vi "Kinesis - MST602 MNA601 - Two Axis Scan.vi"() -> ()   [LabVIEW 2012]
uses:
  U:/Kinesis LabVIEW Website Examples/Thorlabs.MotionControl.Controls.dll
  Thorlabs.MotionControl.Controls.dll
  U:/Kinesis LabVIEW Website Examples/Thorlabs.MotionControl.ModularRackCLI.dll
  Thorlabs.MotionControl.ModularRackCLI.dll
  U:/Kinesis LabVIEW Website Examples/Thorlabs.MotionControl.GenericNanoTrakCLI.dll
  Thorlabs.MotionControl.GenericNanoTrakCLI.dll
  U:/Kinesis LabVIEW Website Examples/Thorlabs.MotionControl.GenericMotorCLI.dll
  Thorlabs.MotionControl.GenericMotorCLI.dll
panel:
  in  "MNA601 Serial Number":string
  in  "MST602 Serial Number":string
  in  "SelectedRange":i32(ring)=3 items=["TIA_Range1_3NA"=3, "TIA_Range2_10NA"=4, "TIA_Range3_30NA"=5, "TIA_Range4_100NA"=6, "TIA_Range5_300NA"=7, "TIA_Range6_1MUA"=8, "TIA_Range7_3MUA"=9, "TIA_Range8_10MUA"=10, "TIA_Range9_30MUA"=11, "TIA_Range10_100MUA"=12, "TIA_Range11_300MUA"=13, "TIA_Range12_1MA"=14, "TIA_Range13_3MA"=15, "TIA_Range14_10MA"=16]
  in  "?":bool
  in  "Num Of Steps":i32=50
  in  "Scale":sgl=0.25 format="%.2f"
  in  "ModularStepperControl Ch.2":refnum<k24>(container)
  in  "ModularStepperControl Ch.1":refnum<k24>(container)
  out "Error":errorcluster
  in  "ModularNanoTrakControl":refnum<k24>(container)
  # "Thorlabs Hardware: \nMST602 Rack Module 2-Ch Stepper Motor Controller \nhttps://www.thorlabs.com/newgrouppage9.cfm?objectgroup_id=1186\n\nMNA601 Rack Module Fiber Auto-alignment Module\nhttps://www.thorlabs.com/newgrouppage9.cfm?objectgroup_id=1187\n\nDescription: The below VI will enable you to connect to a MNA601 & MST602. This VI will initiate a simple 2D raster scan of a Stepper Motor actuated stage. An example of this application setup is pictured whereby the MST602 is driving will drive the internal X & Z piezo blocks of a MAX381 stage. The MAX381 stage is holding an optical fibre aligned to a waveguide in series with secondary receiving fibre via use of Thorlabs flexure stage holder accessories. The secondary fibre is mounted to a secondary co-located MAX302 stage. This fibre is connected to the Optical Input of the MNA601 controller.\n\nThe motorised raster scan will stop either when the max number of steps have been reached or the user selected TIA Range of the MNA601 has been reached, indicating that the MNA601 is reading sufficient photocurrent from the fibre-copupling system. This signifies an \"optimised throughput\" in the system. The MNA601 is defaulted to 'Latch' mode as the MNA601 HV Outputs are not in use.\n\nInstructions: \n1) Connect a MNA601 & MST602 to MMR601 as per the respective product user manuals. These can be connected to any bay in the MMR601 rack.\n2) Enter the module serial numbers below.\n3) Enter the Scan parameters, as well as the exitting TIA Range.\n4) To run the VI, click the run button in the LabVIEW Toolbar.\n5) Once running, the Kinesis UIs will initialise & the VI will wait for you to assign the correct motor types. This can be done by selecting the actuator type on the Kinesis device name on the UI panel & then click 'ACTUATOR SELECTED'\n4) The VI will exit when either the required TIA Range has been reached or the scan has completed."
  # "Notes:"
  # "- Ensure that the appropriate .DLLs are copied into your Project Folder. Check that the correct bit type are used depending on your version of LabVIEW\ni.e. 32-bit or 64-bit.\n\n\n\n\n\n\n\n\n\n\n\n\n\n\n- Open the example VI through the LabVIEW Project Explorer to correctly load the User Interface from Thorlabs.MotionControl.Controls.dll."
  # "Example Image of .NET Controller - VI opened via Project Explorer/ not opened via Project Explorer"
  # "VI Not Opened via Project Explorer"
  # "VI Opened via Project Explorer"
  # "- To explore the range of methods available, please visit the .NET API, included with your Kinesis software.\n\n- For tips on building your own VIs with Thorlabs Motion Control Hardware, please see our LabVIEW Guide here.\nhttps://www.thorlabs.com/newgrouppage9.cfm?objectgroup_id=10285"
  # "52808314"
  # "51810791"
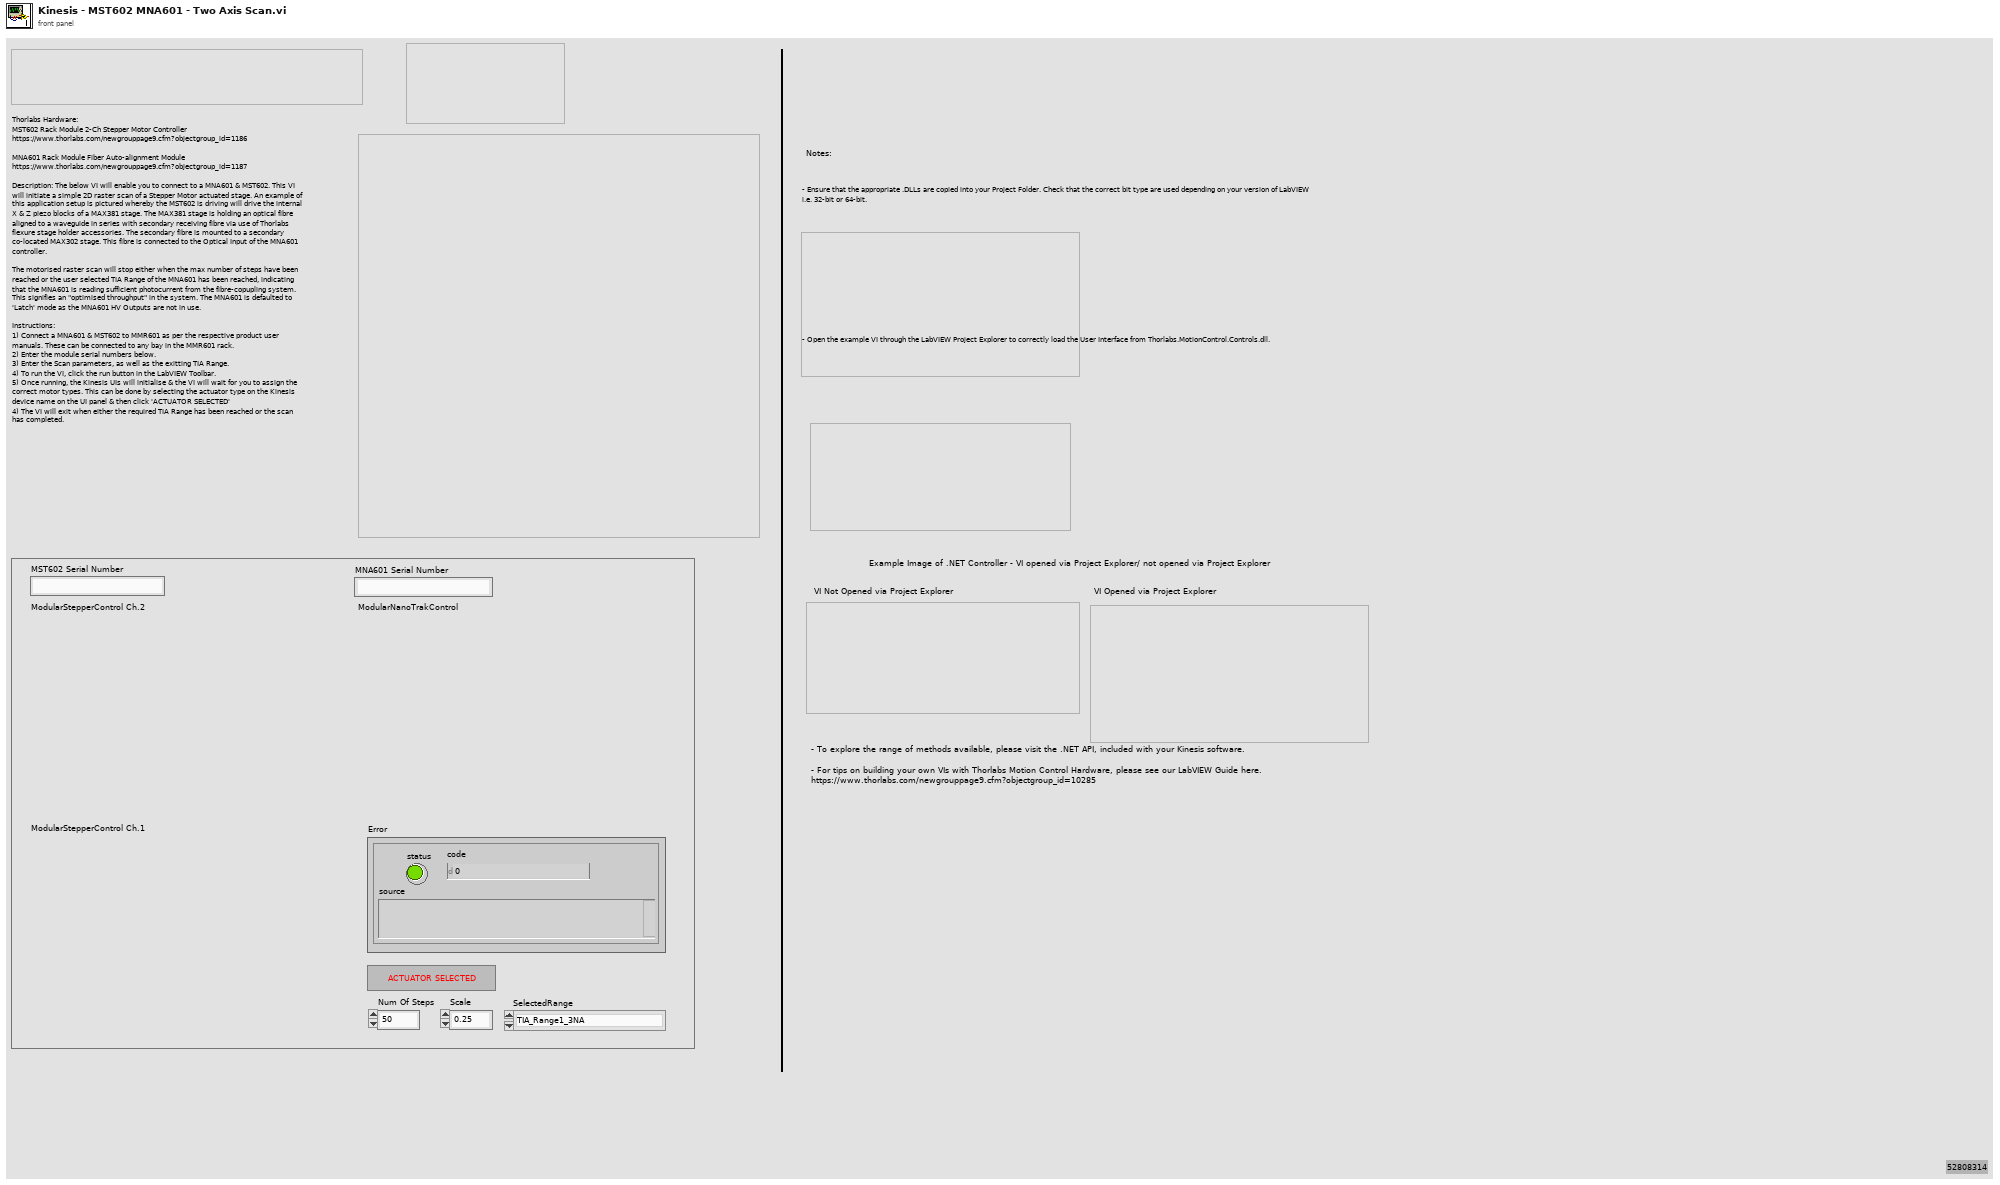
[diagram p1: front panel]
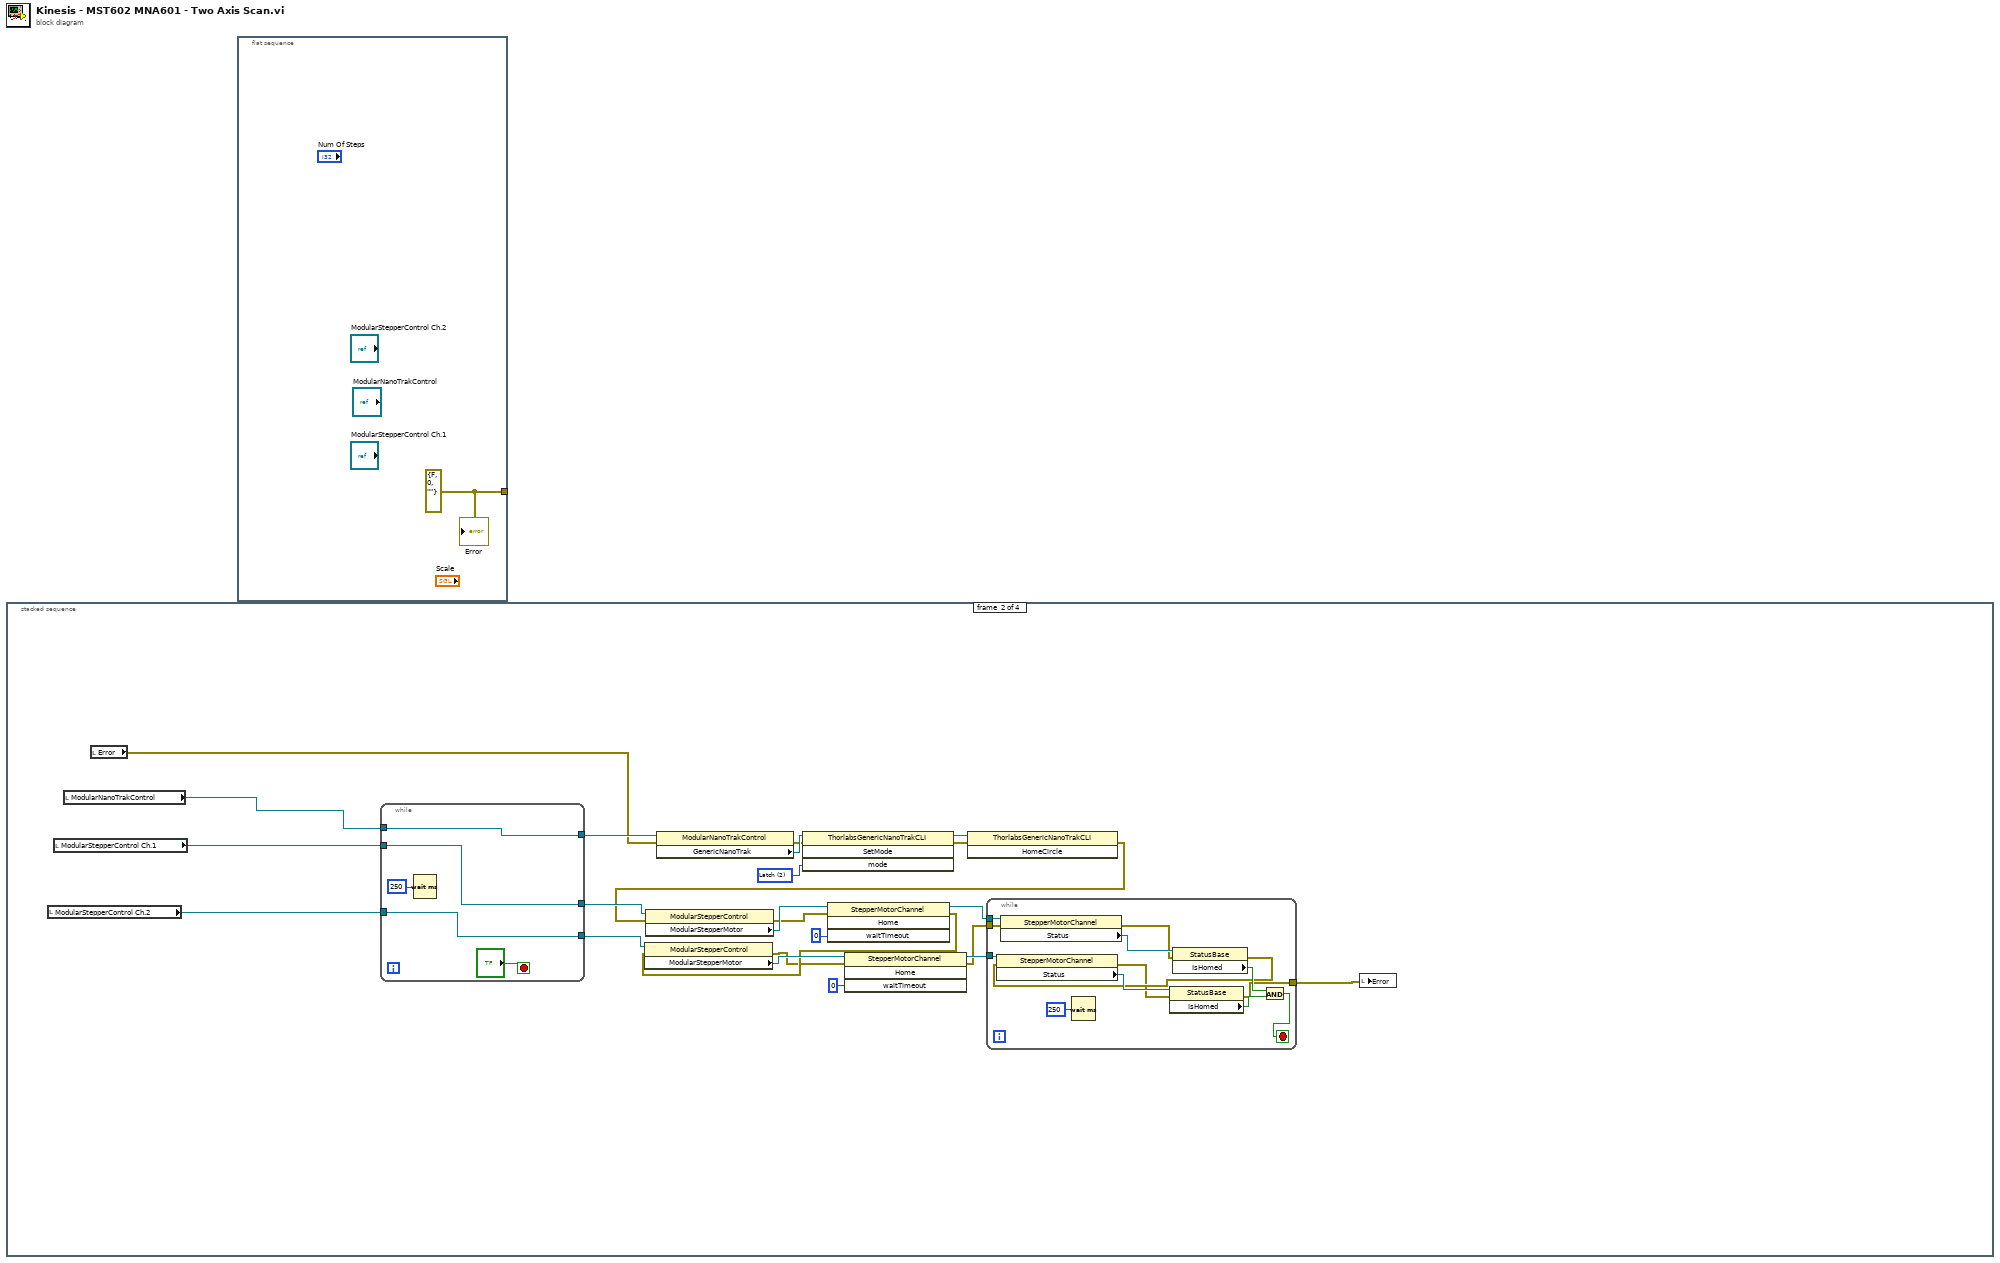
[diagram p0: block diagram]
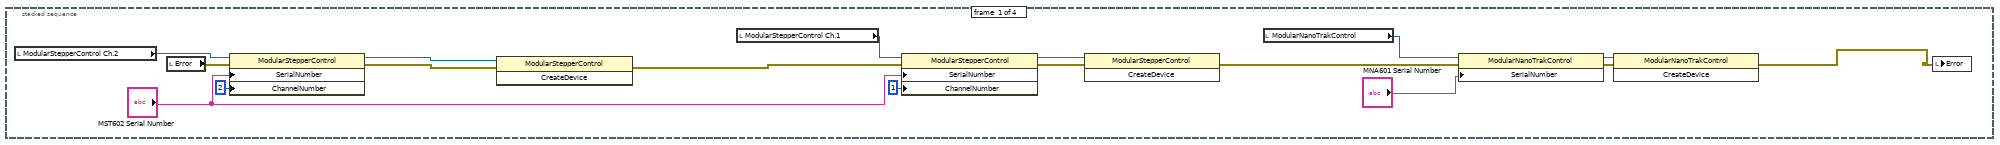
[diagram p2: hidden frame]
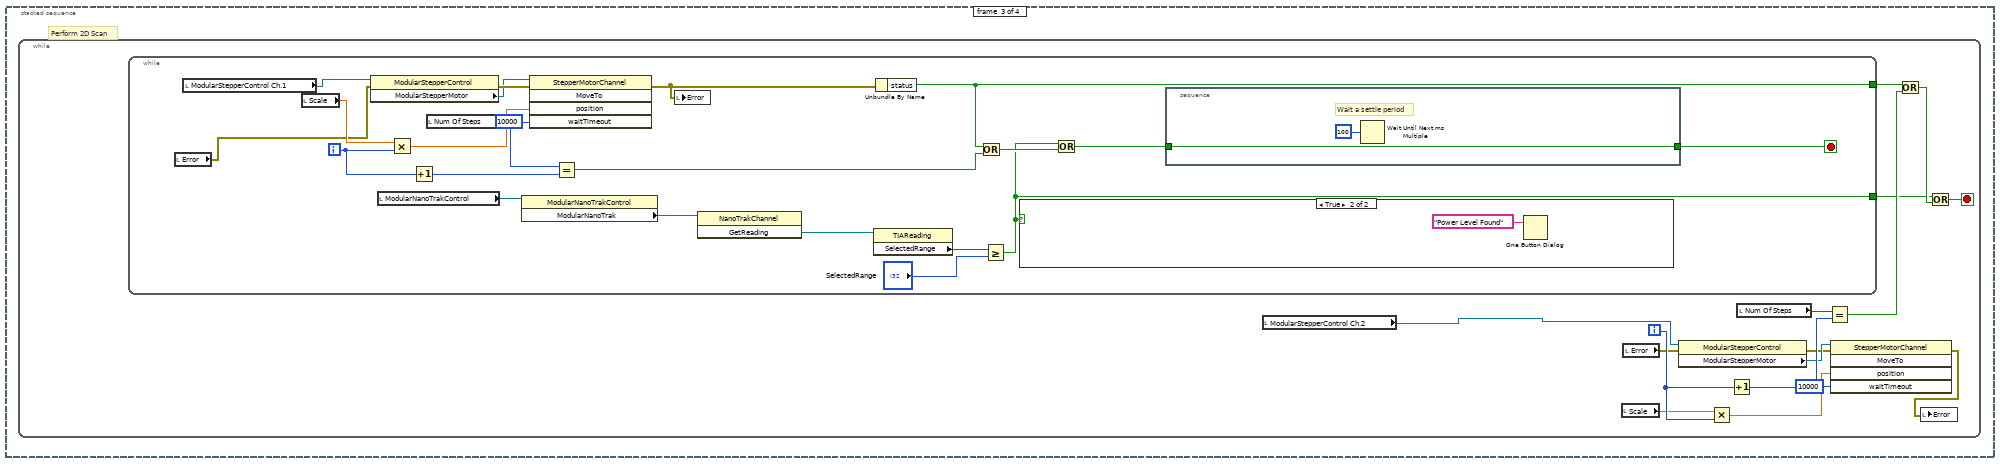
[diagram p3: hidden frame]
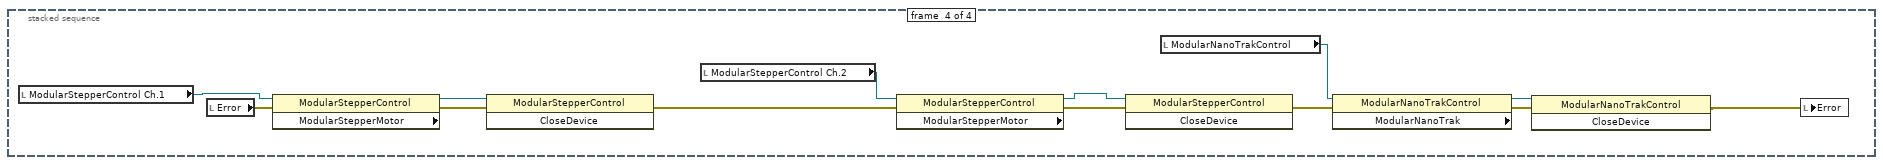
[diagram p5: hidden frame]
diagram:
  n1 = stacked-sequence {
    frame #0 {
      n2 = local read "ModularStepperControl Ch.2"() -> (w7:refnum<k24>)
      n3 = local read "Error"() -> (w14:errorcluster)
      n4 = property class="ModularStepperControl"(reference=w7, error in=w14, "SerialNumber"="MST602 Serial Number", "ChannelNumber"=2) -> (reference out=w17:refnum<k24>, error out=w16:errorcluster)
      n5 = invoke class="ModularStepperControl" method="CreateDevice"(reference=w17, error in=w16) -> (error out=w4:errorcluster)  [unwired: 1 in, 2 out]
      n6 = local read "ModularStepperControl Ch.1"() -> (w6:refnum<k24>)
      n7 = property class="ModularStepperControl"(reference=w6, error in=w4, "SerialNumber"="MST602 Serial Number", "ChannelNumber"=1) -> (reference out=w8:refnum<k24>, error out=w13:errorcluster)
      n8 = invoke class="ModularStepperControl" method="CreateDevice"(reference=w8, error in=w13) -> (error out=w3:errorcluster)  [unwired: 1 in, 2 out]
      n9 = local read "ModularNanoTrakControl"() -> (w11:refnum<k24>)
      n10 = property class="ModularNanoTrakControl"(reference=w11, error in=w3, "SerialNumber"="MNA601 Serial Number") -> (reference out=w10:refnum<k24>, error out=w9:errorcluster)
      n11 = invoke class="ModularNanoTrakControl" method="CreateDevice"(reference=w10, error in=w9) -> (error out=w2:errorcluster)  [unwired: 1 in, 2 out]
      n12 = local write "Error"(w2) -> ()
    }
    frame #1 {
      w37 = 2 items=["Undefined", "Piezo", "Latch", "Tracking", "HorizontalTracking", "VerticalTracking"] ("mode")
      n13 = local read "ModularStepperControl Ch.2"() -> (w33:refnum<k24>)
      n14 = local read "ModularStepperControl Ch.1"() -> (w35:refnum<k24>)
      n15 = local read "ModularNanoTrakControl"() -> (w31:refnum<k24>)
      n16 = local read "Error"() -> (w28:errorcluster)
      n17 = while {
        tunnel: [w58] -> w36
        tunnel: w35 -> [w58]
        tunnel: [w57] -> w34
        tunnel: w33 -> [w57]
        tunnel: [w56] -> w32
        tunnel: w31 -> [w56]
        stop <- "?" stop-if-true
        n18 = Wait (ms)(milliseconds to wait=u32 250) -> ()  [unwired: 1 out]
      }
      n19 = property class="ModularNanoTrakControl"(reference=w32, error in=w28) -> (error out=w39:errorcluster, "GenericNanoTrak"=w41:refnum<k24>)  [unwired: 1 out]
      n20 = invoke class="ThorlabsGenericNanoTrakCLI" method="SetMode"(reference=w41, error in=w39, "mode"=w37) -> (reference out=w40:refnum<k24>, error out=w38:errorcluster)  [unwired: 1 in, 2 out]
      n21 = invoke class="ThorlabsGenericNanoTrakCLI" method="HomeCircle"(reference=w40, error in=w38) -> (error out=w27:errorcluster)  [unwired: 1 in, 2 out]
      n22 = property class="ModularStepperControl"(reference=w36, error in=w27) -> (error out=w26:errorcluster, "ModularStepperMotor"=w30:refnum<k24>)  [unwired: 1 out]
      n23 = invoke class="StepperMotorChannel" method="Home"(reference=w30, error in=w26, "waitTimeout"=0) -> (reference out=w19:refnum<k24>, error out=w25:errorcluster)  [unwired: 1 in, 2 out]
      n24 = property class="ModularStepperControl"(reference=w34, error in=w25) -> (error out=w24:errorcluster, "ModularStepperMotor"=w29:refnum<k24>)  [unwired: 1 out]
      n25 = invoke class="StepperMotorChannel" method="Home"(reference=w29, error in=w24, "waitTimeout"=0) -> (reference out=w21:refnum<k24>, error out=w20:errorcluster)  [unwired: 1 in, 2 out]
      n26 = while {
        tunnel: w21 -> [w54]
        tunnel: w20 -> [w47]
        tunnel: w19 -> [w43]
        tunnel: [w42] -> w18
        stop <- w49 stop-if-true
        n27 = property class="StepperMotorChannel"(reference=w43, error in=w47) -> (error out=w46:errorcluster, "Status"=w52:refnum<k24>)  [unwired: 1 out]
        n28 = Wait (ms)(milliseconds to wait=u32 250) -> ()  [unwired: 1 out]
        n29 = property class="StatusBase"(reference=w52, error in=w46) -> (error out=w45:errorcluster, "IsHomed"=w51:bool)  [unwired: 1 out]
        n30 = property class="StepperMotorChannel"(reference=w54, error in=w45) -> (error out=w44:errorcluster, "Status"=w53:refnum<k24>)  [unwired: 1 out]
        n31 = property class="StatusBase"(reference=w53, error in=w44) -> (error out=w42:errorcluster, "IsHomed"=w50:bool)  [unwired: 1 out]
        n32 = And(x=w51, y=w50) -> (x .and. y?=w49:bool)
      }
      n33 = local write "Error"(w18) -> ()
    }
    frame #2 {
      # "Perform 2D Scan"
      n34 = while {
        i -> [w72]
        stop <- w71 stop-if-true
        n35 = while {
          tunnel: [w92] -> w69
          tunnel: [w96] -> w75
          i -> [w95]
          stop <- w90 stop-if-true
          n36 = local read "Error"() -> (w76:errorcluster)
          n37 = local read "ModularStepperControl Ch.1"() -> (w80:refnum<k24>)
          n38 = local read "Scale"() -> (w81:sgl)
          n39 = property class="ModularStepperControl"(reference=w80, error in=w76) -> (error out=w89:errorcluster, "ModularStepperMotor"=w79:refnum<k24>)  [unwired: 1 out]
          n40 = local read "ModularNanoTrakControl"() -> (w87:refnum<k24>)
          n41 = Multiply(x=w81, y=w95) -> (x*y=w88:sgl)
          n42 = Increment(x=w95) -> (x+1=w94:i32)
          n43 = local read "Num Of Steps"() -> (w82:i32)
          n44 = property class="ModularNanoTrakControl"(reference=w87) -> ("ModularNanoTrak"=w86:refnum<k24>)  [unwired: 1 in, 2 out]
          n45 = invoke class="StepperMotorChannel" method="MoveTo"(reference=w79, error in=w89, "position"=w88, "waitTimeout"=10000) -> (error out=w83:errorcluster)  [unwired: 1 in, 4 out]
          n46 = Equal?(x=w82, y=w94) -> (x = y?=w97:bool)
          n47 = local write "Error"(w83) -> ()
          n48 = invoke class="NanoTrakChannel" method="GetReading"(reference=w86) -> ("GetReading"=w85:refnum<k24>)  [unwired: 2 in, 2 out]
          n49 = property class="TIAReading"(reference=w85) -> ("SelectedRange"=w84:i32)  [unwired: 1 in, 2 out]
          n50 = Unbundle By Name(w83) -> ("status"=w96:bool)
          n51 = Or(x=w96, y=w97) -> (x .or. y?=w93:bool)
          n52 = Greater Or Equal?(x=w84, y="SelectedRange") -> (x >= y?=w92:bool)
          n53 = case shown="True" w92 {
            frame False {
            }
            frame True {
              n54 = One Button Dialog(message="Power Level Found") -> ()  [unwired: 1 in, 1 out]
            }
          }
          n55 = Or(x=w92, y=w93) -> (x .or. y?=w91:bool)
          n56 = stacked-sequence {
            tunnel: w91 -> [w98]
            tunnel: [w98] -> w90
            frame #0 {
              # "Wait a settle period"
              n57 = Wait Until Next ms Multiple(millisecond multiple=u32 100) -> ()  [unwired: 1 out]
            }
          }
        }
        n58 = local read "ModularStepperControl Ch.2"() -> (w62:refnum<k24>)
        n59 = local read "Scale"() -> (w63:sgl)
        n60 = local read "Error"() -> (w66:errorcluster)
        n61 = property class="ModularStepperControl"(reference=w62, error in=w66) -> (error out=w65:errorcluster, "ModularStepperMotor"=w67:refnum<k24>)  [unwired: 1 out]
        n62 = Multiply(x=w63, y=w72) -> (x*y=w68:sgl)
        n63 = Increment(x=w72) -> (x+1=w73:i32)
        n64 = local read "Num Of Steps"() -> (w64:i32)
        n65 = Equal?(x=w64, y=w73) -> (x = y?=w74:bool)
        n66 = invoke class="StepperMotorChannel" method="MoveTo"(reference=w67, error in=w65, "position"=w68, "waitTimeout"=10000) -> (error out=w60:errorcluster)  [unwired: 1 in, 4 out]
        n67 = Or(x=w75, y=w74) -> (x .or. y?=w70:bool)
        n68 = local write "Error"(w60) -> ()
        n69 = Or(x=w69, y=w70) -> (x .or. y?=w71:bool)
      }
    }
    frame #3 {
      n70 = local read "ModularStepperControl Ch.1"() -> (w111:refnum<k24>)
      n71 = local read "Error"() -> (w110:errorcluster)
      n72 = property class="ModularStepperControl" props=["ModularStepperMotor"](reference=w111, error in=w110) -> (reference out=w105:refnum<k24>, error out=w109:errorcluster)  [unwired: 1 out]
      n73 = invoke class="ModularStepperControl" method="CloseDevice"(reference=w105, error in=w109) -> (error out=w108:errorcluster)  [unwired: 1 in, 2 out]
      n74 = local read "ModularStepperControl Ch.2"() -> (w112:refnum<k24>)
      n75 = property class="ModularStepperControl" props=["ModularStepperMotor"](reference=w112, error in=w108) -> (reference out=w104:refnum<k24>, error out=w107:errorcluster)  [unwired: 1 out]
      n76 = invoke class="ModularStepperControl" method="CloseDevice"(reference=w104, error in=w107) -> (error out=w106:errorcluster)  [unwired: 1 in, 2 out]
      n77 = local read "ModularNanoTrakControl"() -> (w113:refnum<k24>)
      n78 = property class="ModularNanoTrakControl" props=["ModularNanoTrak"](reference=w113, error in=w106) -> (reference out=w102:refnum<k24>, error out=w103:errorcluster)  [unwired: 1 out]
      n79 = invoke class="ModularNanoTrakControl" method="CloseDevice"(reference=w102, error in=w103) -> (error out=w101:errorcluster)  [unwired: 1 in, 2 out]
      n80 = local write "Error"(w101) -> ()
    }
  }
  n81 = flat-sequence {
    tunnel: [w114] -> _
    frame #0 {
      w114 = errorcluster {"status"=FALSE, "code"=0, "source"=""} ("Error 2")
      "Error" <- w114
    }
  }
